vi "autobroadsidetimed.vi"() -> ()   [LabVIEW 2012, in "MainProject.lvrbt"]
uses:
  MainProject.lvrbt
  <vilib>/NXT/HiTechnic/HiTechnic Controls/HiTechnic Port.ctl
  <vilib>/NXT/Block Support/NXT_InputPort.ctl
  <vilib>/NXT/Hardware/Plugins/Tetrix DC Motor/TetrixDCMotorAddress.ctl
  <vilib>/NXT/Hardware/Plugins/Tetrix 180 deg Servo/Tetrix180ServoAddress.ctl
  Drivers/AutoDriverControl.ctl
  Drivers/AutoControl3.ctl
  FTC 2012 - 2013/Controls/SpeedControl.ctl
  Drivers/LineCountColorCtl.ctl
  <vilib>/NXT/NXTIO Xnodes/NXTIONodeSubVIs/TETRIX IO Check Battery.vi
  <vilib>/NXT/Dual Mode Library/Waits/Wait_Num(msec).vi
  <vilib>/NXT/NXTIO Xnodes/NXTIONodeSubVIs/TETRIX IO Move Servos.vi
  <vilib>/NXT/NXTIO Xnodes/NXTIONodeSubVIs/TETRIX IO Stop DC Motors.vi
  <vilib>/NXT/Dual Mode Library/Sound/Tone.vi
  <vilib>/NXT/Dual Mode Library/Waits/Wait_Num.vi
  <vilib>/NXT/Subs/LVHSConnector.ctl
  <vilib>/NXT/NXTIO Xnodes/AddressXNode/NXTIOAddress.xnode
  <vilib>/NXT/NXTIO Xnodes/NXTIOXNode/NXTIO.xnode
  <vilib>/NXT/LegoClasses/BrickReference/BrickReference.lvclass
panel:
  out "Color":string="Black"
  out "Sector (0-9)":i16
  out "Enabled":bool
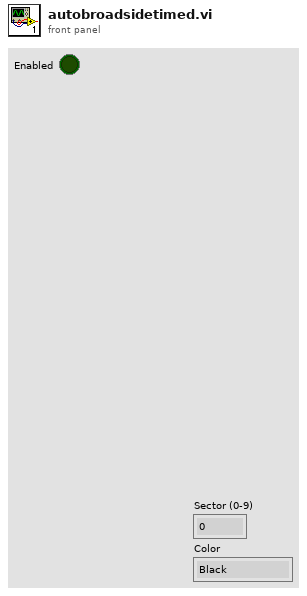
[diagram p1: front panel]
types:
  T1 = typedef "HiTechnic Port.ctl" = cluster{"Port":T2, "MUX Port":u8}
  T2 = typedef "NXT_InputPort.ctl" = u8
  T3 = typedef "TetrixDCMotorAddress.ctl" = i16
  T4 = typedef "LVHSConnector.ctl" = refnum<class "BrickReference.lvclass">
  T5 = typedef "Tetrix180ServoAddress.ctl" = i16
  T6 = typedef "AutoDriverControl.ctl" = enum16{"Init", "Forward", "Reverse", "Left", "Right", "Brake"}
  T7 = typedef "AutoControl3.ctl" = enum16{"FindIRBasket", "DropBLK", "DrvToEndOfBaskets", "DrvAroundBaskets", "AlignWithRamp", "ParkOnRamp", "Stop"}
  T8 = cluster{"Tetrix180Servo":T5, "Tetrix180Servo 2":T5, "Tetrix180Servo 3":T5, "Tetrix180Servo 4":T5}
  T9 = typedef "LineCountColorCtl.ctl" = enum16{"Init/Reset", "Check"}
  T10 = typedef "SpeedControl.ctl" = enum16{"Fast", "Medium", "Slow"}
  T11 = cluster{"Tetrix180Servo":T5, "Tetrix180Servo":T5, "Tetrix180Servo":T5, "Tetrix180Servo":T5}
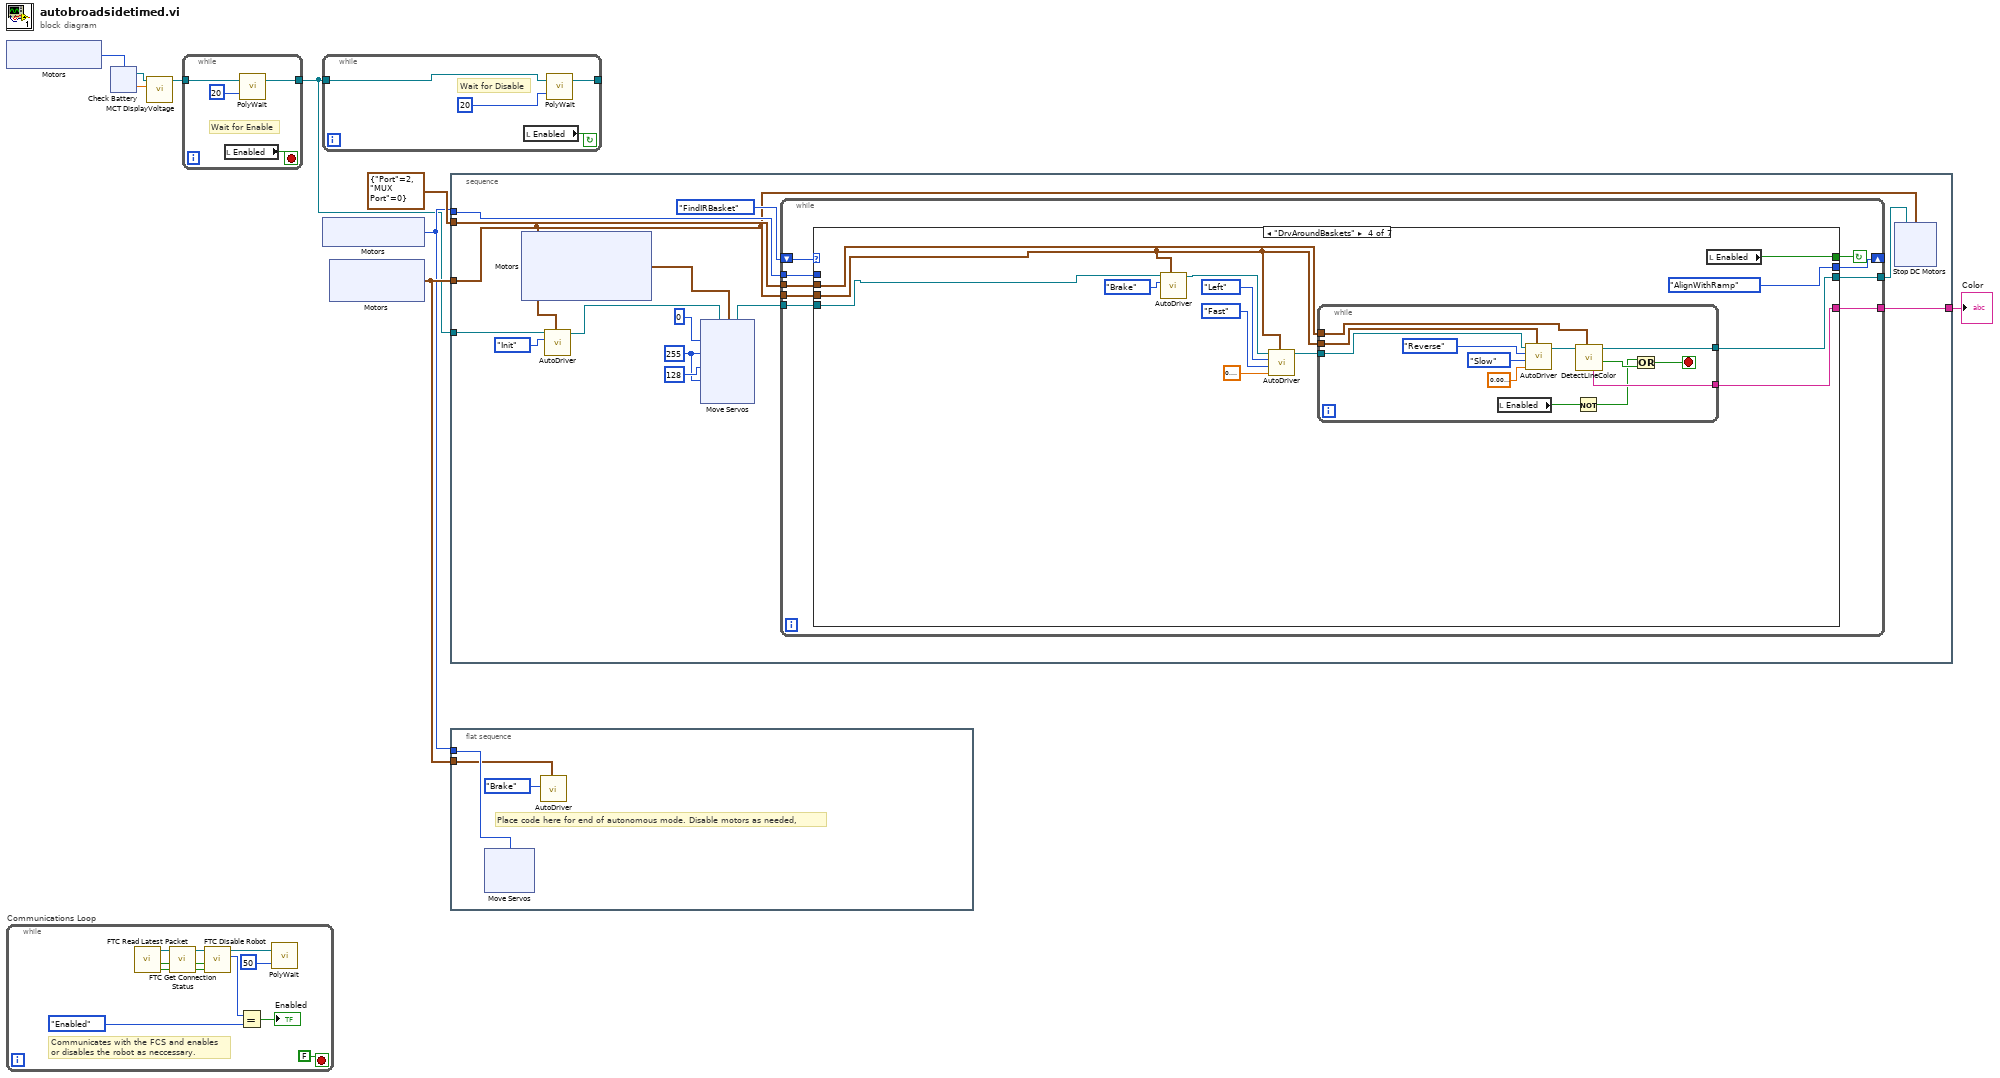
[diagram p0: block diagram]
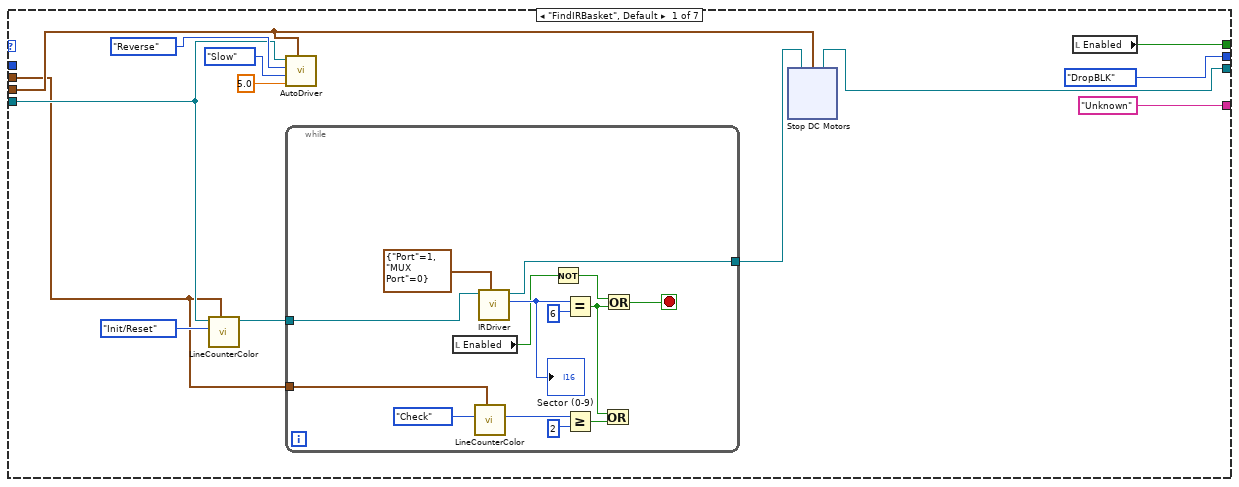
[diagram p2: hidden frame]
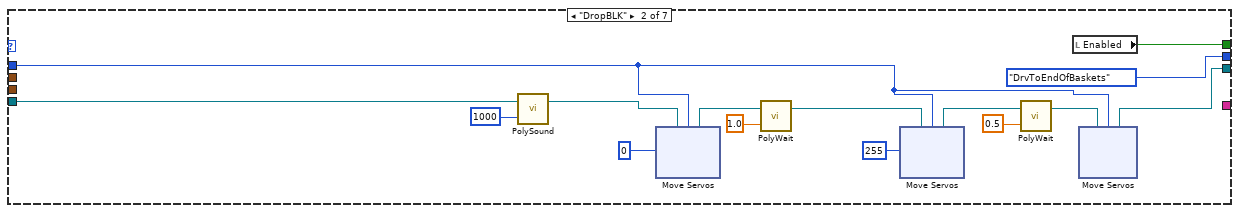
[diagram p3: hidden frame]
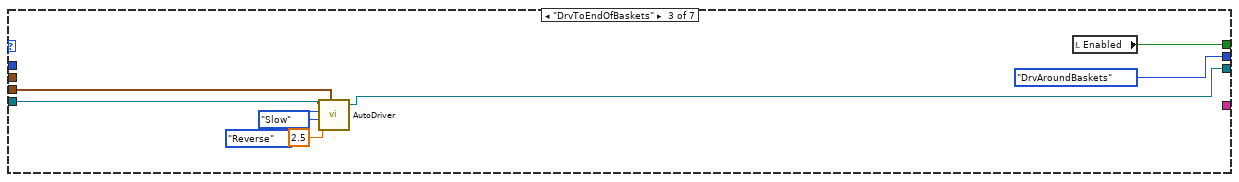
[diagram p4: hidden frame]
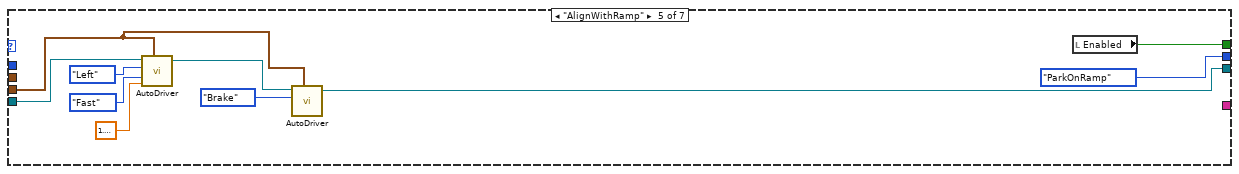
[diagram p5: hidden frame]
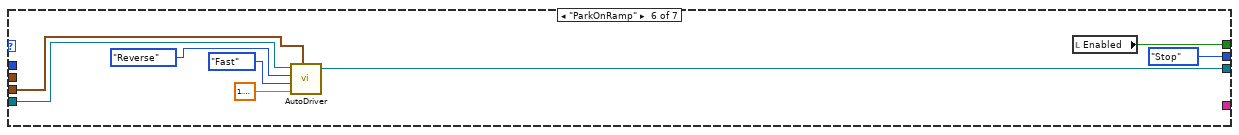
[diagram p6: hidden frame]
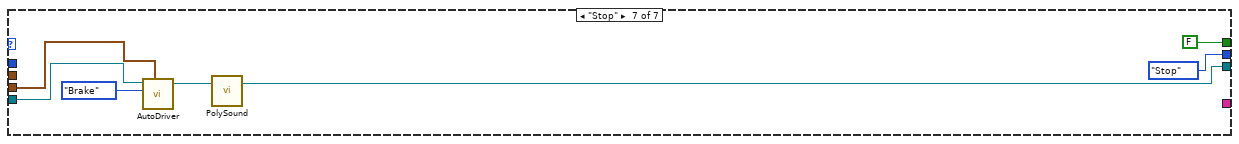
[diagram p7: hidden frame]
diagram:
  n1 = xnode "Motors"() -> ("Motor"=w4:T3)
  n2 = while "Communications Loop" {
    stop <- FALSE stop-if-true
    # "Communicates with the FCS and enables \nor disables the robot as neccessary."
    n3 = call <vilib>:"FTC Read Latest Packet.vi"() -> ("Packet Received?"=w19:bool, "Stopped?"=w18:bool, "NXT"=w21:T4)  [unwired: 6 in, 3 out]
    n4 = call <vilib>:"FTC Get Connection Status.vi"("Packet Received?"=w19, "Stopped?"=w18, "NXT"=w21) -> ("Online?"=w11:bool, "Stopped?"=w12:bool, "NXT"=w20:T4)  [unwired: 5 in]
    n5 = call <vilib>:"FTC Disable Robot.vi"("Online?"=w11, "Stopped?"=w12, "NXT"=w20) -> ("Enabled?"=w14:enum16{"Disabled", "Enabled"}, "NXT"=w16:T4)  [unwired: 3 in]
    n6 = Equal?(x=w14, y=enum16{"Disabled", "Enabled"}."Enabled") -> (x = y?=→"Enabled":bool)
    n7 = call-poly <vilib>:"PolyWait.vi"("Time (100 msec)"=u32 50 ("Time (msec)"), "NXT"=w16) -> ()  [unwired: 2 in, 1 out]
  }
  n8 = xnode "Check Battery"("Motors"=w4) -> ("Voltage 1"=w8:sgl, "NXT"=w9:T4)  [unwired: 1 in]
  n9 = call <vilib>:"MCT DisplayVoltage.vi"("Motor Voltage"=w8, "NXT"=w9) -> ("NXT"=w7:T4)  [unwired: 9 in]
  n10 = while {
    tunnel: [w24] -> w1
    tunnel: w7 -> [w22]
    stop <- w23 stop-if-true
    # "Wait for Enable"
    n11 = local read "Enabled"() -> (w23:bool)
    n12 = call-poly <vilib>:"PolyWait.vi"("Time (100 msec)"=u32 20 ("Time (msec)"), "NXT"=w22) -> ("NXT"=w24:T4)  [unwired: 2 in]
  }
  n13 = while {
    tunnel: [w27] -> _
    tunnel: w1 -> [w26]
    stop <- w28 continue-if-true
    # "Wait for Disable"
    n14 = local read "Enabled"() -> (w28:bool)
    n15 = call-poly <vilib>:"PolyWait.vi"("Time (100 msec)"=u32 20 ("Time (msec)"), "NXT"=w26) -> ("NXT"=w27:T4)  [unwired: 2 in]
  }
  n16 = xnode "Motors"() -> ("Motor"=w3:T5)
  n17 = xnode "Motors"() -> ("Motor"=w6:cluster{"TetrixDCMotor":T3, "TetrixDCMotor":T3})
  n18 = stacked-sequence {
    tunnel: w6 -> [w36]
    tunnel: w1 -> [w41]
    tunnel: T1 {"Port"=2, "MUX Port"=0} ("Port/MUX") -> [w42]
    tunnel: w3 -> [w38]
    tunnel: [w37] -> w2
    frame #0 {
      w30 = u8 255 ("Position 2")
      n19 = xnode "Motors"() -> ("Motor"=w33:T11)
      n20 = call "AutoDriver.vi"("NXT In"=w41, "Motors"=w36, "Direction"=AutoDriverControl."Init") -> ("NXT Out"=w40:T4)  [unwired: 5 in]
      n21 = xnode "Move Servos"("Position 4"=w30, "Position 3"=u8 128 ("Position 5"), "Position 2"=w30, "Position 1"=u8 0, "Servos"=w33, "NXT"=w40) -> ("NXT"=w34:T4)
      n22 = while {
        tunnel: w36 -> [w74]
        tunnel: w34 -> [w73]
        shift-right: [w72] -> _
        shift-left: AutoControl3."FindIRBasket" -> [w71]
        tunnel: w42 -> [w70]
        tunnel: w38 -> [w68]
        tunnel: [w67] -> w37
        tunnel: [w66] -> w35
        stop <- w69 continue-if-true
        n23 = case shown="\"DrvAroundBaskets\"" w71 {
          tunnel: w74 -> [w82 _ w148 w158 w180 w195 w203]
          tunnel: w73 -> [w83 w115 w150 w153 w179 w196 w202]
          tunnel: [AutoControl3."DropBLK" AutoControl3."DrvToEndOfBaskets" AutoControl3."DrvAroundBaskets" AutoControl3."AlignWithRamp" AutoControl3."ParkOnRamp" AutoControl3."Stop" AutoControl3."Stop"] -> w72
          tunnel: w70 -> [w75 _ _ w161 _ _ _]
          tunnel: [w79 w114 w151 w155 w182 w190 FALSE] -> w69
          tunnel: w68 -> [_ w109 _ _ _ _ _]
          tunnel: ["Unknown" ("Color") _ _ w156 _ _ _] -> w67
          tunnel: [w78 w113 w149 w154 w181 w189 w197] -> w66
          frame "FindIRBasket", Default {
            n24 = call "LineCounterColor.vi"("Port/MUX"=w75, "Enum"=LineCountColorCtl."Init/Reset", "NXT In"=w83) -> ("NXT Out"=w77:T4)  [unwired: 7 in, 1 out]
            n25 = call "AutoDriver.vi"("NXT In"=w83, "Motors"=w82, "Direction"=AutoDriverControl."Reverse", "Speed"=SpeedControl."Slow", "Time (1 sec)"=sgl 5.0) -> ()  [unwired: 3 in, 1 out]
            n26 = while {
              tunnel: w77 -> [w105]
              tunnel: w75 -> [w101]
              tunnel: [w102] -> w80
              stop <- w98 stop-if-true
              n27 = local read "Enabled"() -> (w99:bool)
              n28 = call "LineCounterColor.vi"("Port/MUX"=w101, "Enum"=LineCountColorCtl."Check") -> ("Numeric"=w96:i16)  [unwired: 8 in, 1 out]
              n29 = call "IRDriver.vi"("Port"=T1 {"Port"=1, "MUX Port"=0}, "NXT In"=w105) -> ("Sector (0-9)"=w107:i16, "NXT Out"=w102:T4)  [unwired: 8 in]
              "Sector (0-9)" <- w107
              n30 = Not(x=w99) -> (.not. x?=w97:bool)
              n31 = Equal?(x=w107, y=i16 6) -> (x = y?=w95:bool)
              n32 = Greater Or Equal?(x=w96, y=i16 2) -> (x >= y?=w103:bool)
              n33 = Or(x=w95, y=w103) -> ()  [unwired: 1 out]
              n34 = Or(x=w97, y=w95) -> (x .or. y?=w98:bool)
            }
            n35 = xnode "Stop DC Motors"("Motors"=w82, "NXT"=w80) -> ("NXT"=w78:T4)
            n36 = local read "Enabled"() -> (w79:bool)
          }
          frame "DropBLK" {
            n37 = call-poly <vilib>:"PolySound.vi"("Duration (500 ms)"=u16 1000, "NXT"=w115) -> ("NXT"=w111:T4)  [unwired: 2 in]
            n38 = xnode "Move Servos"("Position 1"=u8 0, "Servos"=w109, "NXT"=w111) -> ("NXT"=w110:T4)
            n39 = call-poly <vilib>:"PolyWait.vi"("Time (1 sec)"=sgl 1.0, "NXT"=w110) -> ("NXT"=w120:T4)  [unwired: 2 in]
            n40 = xnode "Move Servos"("Position 1"=u8 255, "Servos"=w109, "NXT"=w120) -> ("NXT"=w119:T4)
            n41 = call-poly <vilib>:"PolyWait.vi"("Time (1 sec)"=sgl 0.5, "NXT"=w119) -> ("NXT"=w116:T4)  [unwired: 2 in]
            n42 = local read "Enabled"() -> (w114:bool)
            n43 = xnode "Move Servos"("Servos"=w109, "NXT"=w116) -> ("NXT"=w113:T4)  [unwired: 1 in]
          }
          frame "DrvToEndOfBaskets" {
            n44 = call "AutoDriver.vi"("NXT In"=w150, "Motors"=w148, "Direction"=AutoDriverControl."Reverse", "Speed"=SpeedControl."Slow", "Time (1 sec)"=sgl 2.5) -> ("NXT Out"=w149:T4)  [unwired: 3 in]
            n45 = local read "Enabled"() -> (w151:bool)
          }
          frame "DrvAroundBaskets" {
            n46 = call "AutoDriver.vi"("NXT In"=w153, "Motors"=w158, "Direction"=AutoDriverControl."Brake") -> ("NXT Out"=w159:T4)  [unwired: 5 in]
            n47 = call "AutoDriver.vi"("NXT In"=w159, "Motors"=w158, "Direction"=AutoDriverControl."Left", "Speed"=SpeedControl."Fast", "Time (1 sec)"=sgl 0.8) -> ("NXT Out"=w162:T4)  [unwired: 3 in]
            n48 = while {
              tunnel: w158 -> [w178]
              tunnel: w162 -> [w177]
              tunnel: w161 -> [w172]
              tunnel: [w171] -> w156
              tunnel: [w170] -> w154
              stop <- w167 stop-if-true
              n49 = local read "Enabled"() -> (w169:bool)
              n50 = call "AutoDriver.vi"("NXT In"=w177, "Motors"=w178, "Direction"=AutoDriverControl."Reverse", "Speed"=SpeedControl."Slow", "Time (1 sec)"=sgl 0.01) -> ("NXT Out"=w173:T4)  [unwired: 3 in]
              n51 = Not(x=w169) -> (.not. x?=w166:bool)
              n52 = call "DetectLineColor.vi"("Port/MUX"=w172, "NXT In"=w173) -> ("Detected Line?"=w168:bool, "NXT Out"=w170:T4, "Color"=w171:string)  [unwired: 7 in]
              n53 = Or(x=w166, y=w168) -> (x .or. y?=w167:bool)
            }
            n54 = local read "Enabled"() -> (w155:bool)
          }
          frame "AlignWithRamp" {
            n55 = call "AutoDriver.vi"("NXT In"=w179, "Motors"=w180, "Direction"=AutoDriverControl."Left", "Speed"=SpeedControl."Fast", "Time (1 sec)"=sgl 1.1) -> ("NXT Out"=w184:T4)  [unwired: 3 in]
            n56 = call "AutoDriver.vi"("NXT In"=w184, "Motors"=w180, "Direction"=AutoDriverControl."Brake") -> ("NXT Out"=w181:T4)  [unwired: 5 in]
            n57 = local read "Enabled"() -> (w182:bool)
          }
          frame "ParkOnRamp" {
            n58 = call "AutoDriver.vi"("NXT In"=w196, "Motors"=w195, "Direction"=AutoDriverControl."Reverse", "Speed"=SpeedControl."Fast", "Time (1 sec)"=sgl 1.3) -> ("NXT Out"=w189:T4)  [unwired: 3 in]
            n59 = local read "Enabled"() -> (w190:bool)
          }
          frame "Stop" {
            n60 = call "AutoDriver.vi"("NXT In"=w202, "Motors"=w203, "Direction"=AutoDriverControl."Brake") -> ("NXT Out"=w200:T4)  [unwired: 5 in]
            n61 = call-poly <vilib>:"PolySound.vi"("NXT"=w200) -> ("NXT"=w197:T4)  [unwired: 3 in]
          }
        }
      }
      n62 = xnode "Stop DC Motors"("Motors"=w36, "NXT"=w35) -> ()  [unwired: 1 out]
    }
  }
  "Color" <- w2
  n63 = flat-sequence {
    tunnel: w6 -> [w205]
    tunnel: w3 -> [w206]
    frame #0 {
      # "Place code here for end of autonomous mode. Disable motors as needed,"
      n64 = xnode "Move Servos"("Servos"=w206) -> ()  [unwired: 2 in, 1 out]
      n65 = call "AutoDriver.vi"("Motors"=w205, "Direction"=AutoDriverControl."Brake") -> ()  [unwired: 6 in, 1 out]
    }
  }
